vi "CalculatePower.vi"(6 "Reset":bool, 9 "Process Variables":cluster{"Pos":dbl, "Vel":dbl, "Accel":dbl}, 10 "Constants":T1={"FF"=0.009, "AFF"=0.002, "PID gains"={"P"=0.07, "I"=0.0, "D"=0.0}} {"PID gains"."D" format="%.3f"; "PID gains"."I" format="%.3f"; "PID gains"."P" format="%.3f"}, 11 "Setpoints":cluster{"Pos":dbl, "Vel":dbl, "Accel":dbl}) -> (3 "Power":dbl)   [LabVIEW 2016]
uses:
  <vilib>/addons/control/pid/pid.llb/PID (DBL).vi
  <vilib>/addons/control/pid/NI_PID_pid.lvlib
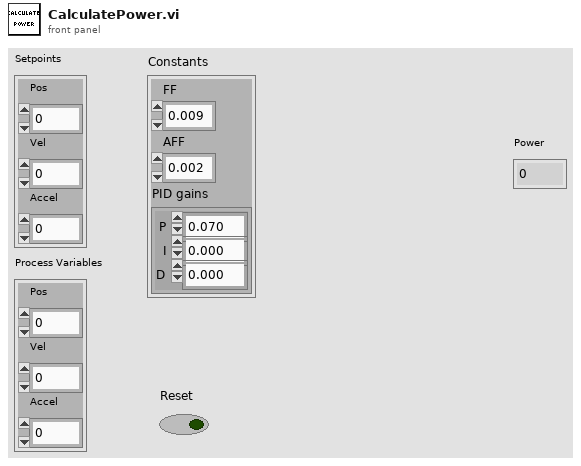
[diagram p1: front panel]
types:
  T1 = cluster{"FF":dbl, "AFF":dbl, "PID gains":cluster{"P":dbl, "I":dbl, "D":dbl}}
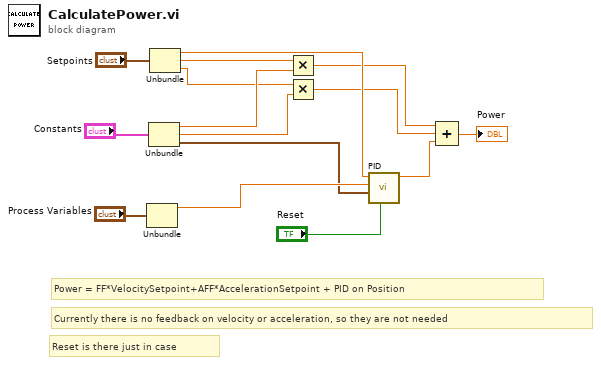
[diagram p0: block diagram]
diagram:
  # "Currently there is no feedback on velocity or acceleration, so they are not needed"
  # "Reset is there just in case"
  # "Power = FF*VelocitySetpoint+AFF*AccelerationSetpoint + PID on Position"
  n1 = Unbundle("Process Variables") -> ("Pos"=w12:dbl)  [unwired: 2 out]
  n2 = Unbundle("Constants") -> ("FF"=w9:dbl, "AFF"=w7:dbl, "PID gains"=w11:cluster{"P":dbl, "I":dbl, "D":dbl})
  n3 = Unbundle("Setpoints") -> ("Pos"=w10:dbl, "Vel"=w8:dbl, "Accel"=w6:dbl)
  n4 = Multiply(x=w8, y=w9) -> (x*y=w1:dbl)
  n5 = Multiply(x=w6, y=w7) -> (x*y=w2:dbl)
  n6 = call-poly <vilib>:"PID.vi"("reinitialize? (F)"="Reset", "PID gains"=w11, "process variable"=w12, "setpoint"=w10) -> ("output"=w5:dbl)  [unwired: 6 in, 1 out]
  n7 = Compound Arithmetic op=ADD(w1, w2, w5) -> (→"Power":dbl)
